vi "Subdivide.vi"(8 "Minimum":dbl, 9 "Maximum":dbl, 10 "Params":T1={"Duration (s)"=0.3, "offset (s)"=0.001, "Threshold"=0.2763157894736842, "Positions"=12, "Taps/Position"=5, "set name"="", "freq res"=5} {"Threshold" scale=0.0..1.0}, 11 "Waveform Graph":waveform(dbl)[](graph)) -> (1 "duration (pts)":dbl, 2 "Array":dbl[](array[numeric]), 3 "Waveform Graph 2":waveform(dbl)[](graph))   [LabVIEW 2022 SP3]
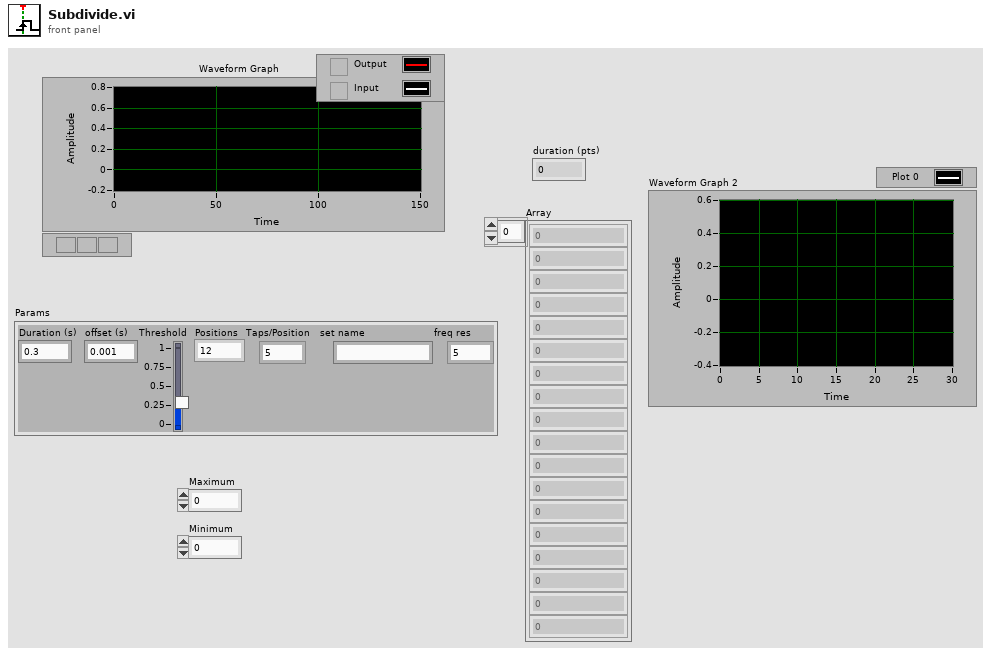
[diagram p1: front panel]
types:
  T1 = cluster{"Duration (s)":dbl, "offset (s)":dbl, "Threshold":dbl, "Positions":i16, "Taps/Position":i16, "set name":string, "freq res":i16}
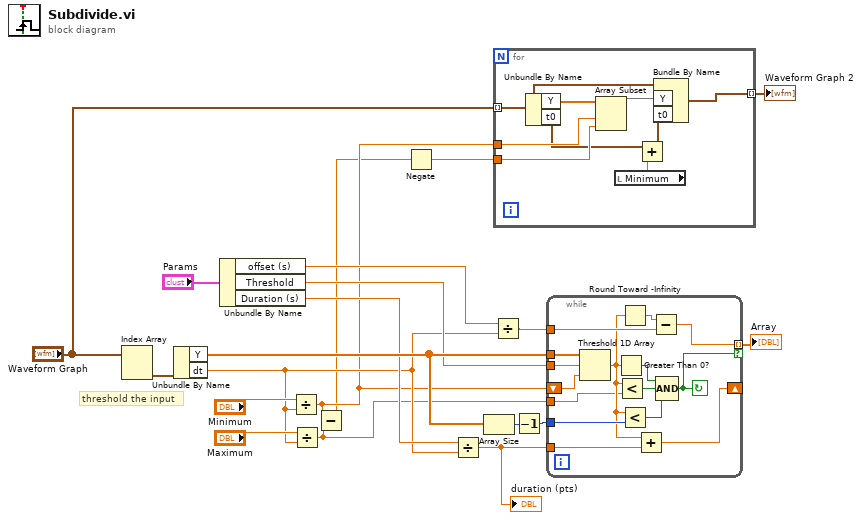
[diagram p0: block diagram]
diagram:
  # "threshold the input"
  n1 = Index Array(array="Waveform Graph") -> (element #2=w8:waveform(dbl))  [unwired: 2 in, 1 out]
  n2 = Unbundle By Name(w8) -> ("Y"=w15:dbl[], "dt"=w6:dbl)
  n3 = Unbundle By Name("Params") -> ("offset (s)"=w20:dbl, "Threshold"=w12:dbl, "Duration (s)"=w11:dbl)
  n4 = Divide(x="Minimum", y=w6) -> (x/y=w5:dbl)
  n5 = Divide(x="Maximum", y=w6) -> (x/y=w4:dbl)
  n6 = Subtract(x=w5, y=w4) -> (x-y=w3:dbl)
  n7 = Negate(x=w3) -> (-x=w1:dbl)
  n8 = Divide(x=w11, y=w6) -> (x/y=w17:dbl)
  "duration (pts)" <- w17
  n9 = Array Size(array=w15) -> (size(s)=w14:i32)
  n10 = Divide(x=w20, y=w6) -> (x/y=w18:dbl)
  n11 = for {
    tunnel: "Waveform Graph" -> [w26] mode=indexing
    tunnel: w5 -> [w28]
    tunnel: w1 -> [w27]
    tunnel: [w24] -> w2 mode=indexing
    n12 = Unbundle By Name(w26) -> ("Y"=w29:dbl[], "t0"=w23:timestamp)
    n13 = Array Subset(array=w29, index=w28, length=w27) -> (w25:dbl[])
    n14 = local read "Minimum"() -> (w22:dbl)
    n15 = Add(x=w23, y=w22) -> (x+y=w21:timestamp)
    n16 = Bundle By Name(cluster=w26, "Y"=w25, "t0"=w21) -> (w24:waveform(dbl))
  }
  "Waveform Graph 2" <- w2
  n17 = Decrement(x=w14) -> (x-1=w13:i32)
  n18 = while {
    tunnel: w15 -> [w44]
    tunnel: w12 -> [w43]
    shift-right: [w39] -> _
    shift-left: w5 -> [w38]
    tunnel: [w31] -> w16 mode=indexing if=w35
    tunnel: w17 -> [w42]
    tunnel: w18 -> [w40]
    tunnel: w4 -> [w30]
    tunnel: w13 -> [w34]
    stop <- w35 continue-if-true
    n19 = Threshold 1D Array(1:w38, 2:w43, 3:w44) -> (0:w32:dbl)
    n20 = Greater Than 0?(x=w32) -> (x > 0?=w36:bool)
    n21 = Less?(x=w32, y=w30) -> (x < y?=w37:bool)
    n22 = Round Toward -Infinity(1:w32) -> (0:w41:dbl)
    n23 = Less?(x=w32, y=w34) -> (x < y?=w33:bool)
    n24 = Add(x=w32, y=w42) -> (x+y=w39:dbl)
    n25 = Subtract(x=w41, y=w40) -> (x-y=w31:dbl)
    n26 = Compound Arithmetic op=AND(w36, w37, w33) -> (w35:bool)
  }
  "Array" <- w16
